vi "SequenceIndexDelete.vi"(8 "error in (no error)":errorcluster, 10 "SequenceIndexName":string, 11 "VariableManager in":refnum<class "VariableManager.lvclass">) -> (0 "error out":errorcluster, 3 "VariableManager out":refnum<class "VariableManager.lvclass">)   [LabVIEW 2013, in "VariableManager.lvclass"]
doc: "Delete SequenceIndexName from database. \nNo operation if SequenceIndexName does not exist"
uses:
  VariableManager.lvclass
  SequenceIndex/SequenceIndex.lvclass
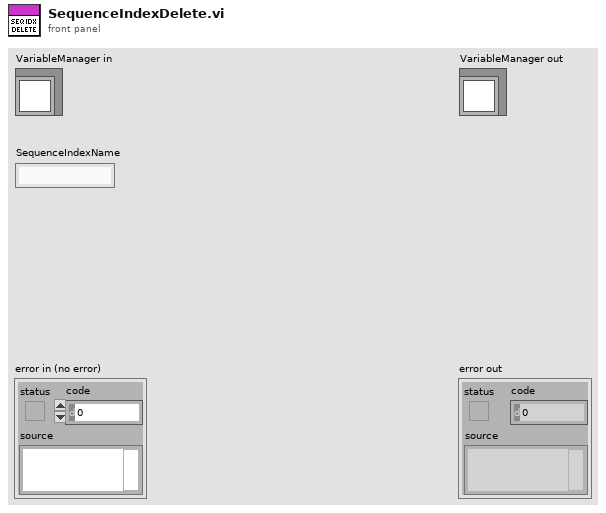
[diagram p1: front panel]
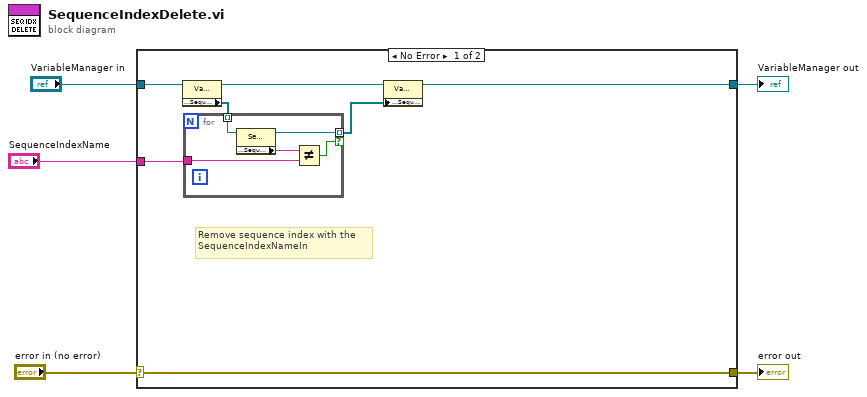
[diagram p0: block diagram]
diagram:
  n1 = case shown="No Error" "error in (no error)" {
    selector: "error in (no error)" -> [w12 w19]
    tunnel: [w12 w19] -> w4
    tunnel: [w7 w18] -> w2
    tunnel: "VariableManager in" -> [w8 w18]
    tunnel: "SequenceIndexName" -> [w6 _]
    frame No Error {
      # "Remove sequence index with the\nSequenceIndexNameIn"
      n2 = property class="VariableManager.lvclass"(reference=w8) -> (reference out=w10:refnum<class "VariableManager.lvclass">, "Accessors:SequenceIndices"=w9:refnum<class "SequenceIndex.lvclass">[])  [unwired: 1 in, 1 out]
      n3 = for {
        tunnel: w9 -> [w17] mode=indexing
        tunnel: w6 -> [w14]
        tunnel: [w16] -> w11 mode=indexing if=w13
        n4 = property class="SequenceIndex.lvclass"(reference=w17) -> (reference out=w16:refnum<class "SequenceIndex.lvclass">, "Accessors:SequenceIndexName"=w15:string)  [unwired: 1 in, 1 out]
        n5 = Not Equal?(x=w15, y=w14) -> (x != y?=w13:bool)
      }
      n6 = property class="VariableManager.lvclass"(reference=w10, "Accessors:SequenceIndices"=w11) -> (reference out=w7:refnum<class "VariableManager.lvclass">)  [unwired: 1 in, 1 out]
    }
    frame Error {
    }
  }
  "error out" <- w4
  "VariableManager out" <- w2
